vi "Poke-n-probe position.vi"(6 "Tries":i32=150, 7 "Goal":T1, 8 "error in":errorcluster, 9 "Speed":dbl=10.0, 10 "Zone":dbl=5.0 caption="mm", 11 "Location":string="Base") -> (0 "error out":errorcluster, 1 "Speed Out":dbl, 2 "Success":bool, 3 "Location Out":string="Base", 5 "Pose":T1)   [LabVIEW 2013]
uses:
  ROS/Code/Console/Servers/ServerSubs/(nist) Arm Globals.vi
panel:
  out "Array":dbl[][](array[numeric])
  out "Try":i32
  in  "stop":bool
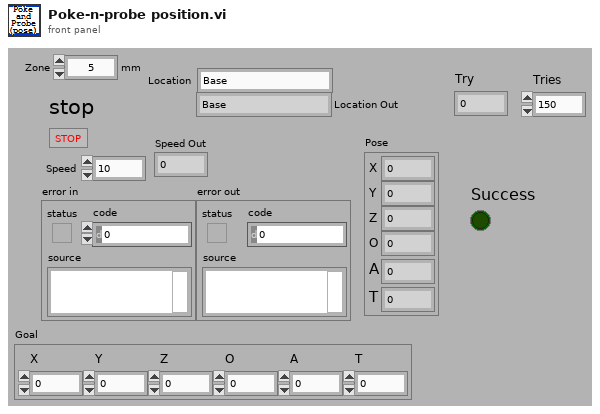
[diagram p1: front panel]
types:
  T1 = cluster{"X":dbl, "Y":dbl, "Z":dbl, "O":dbl, "A":dbl, "T":dbl}
  T2 = typedef "NI_Matrix.lvlib/RealMatrix.ctl" = dbl[][]
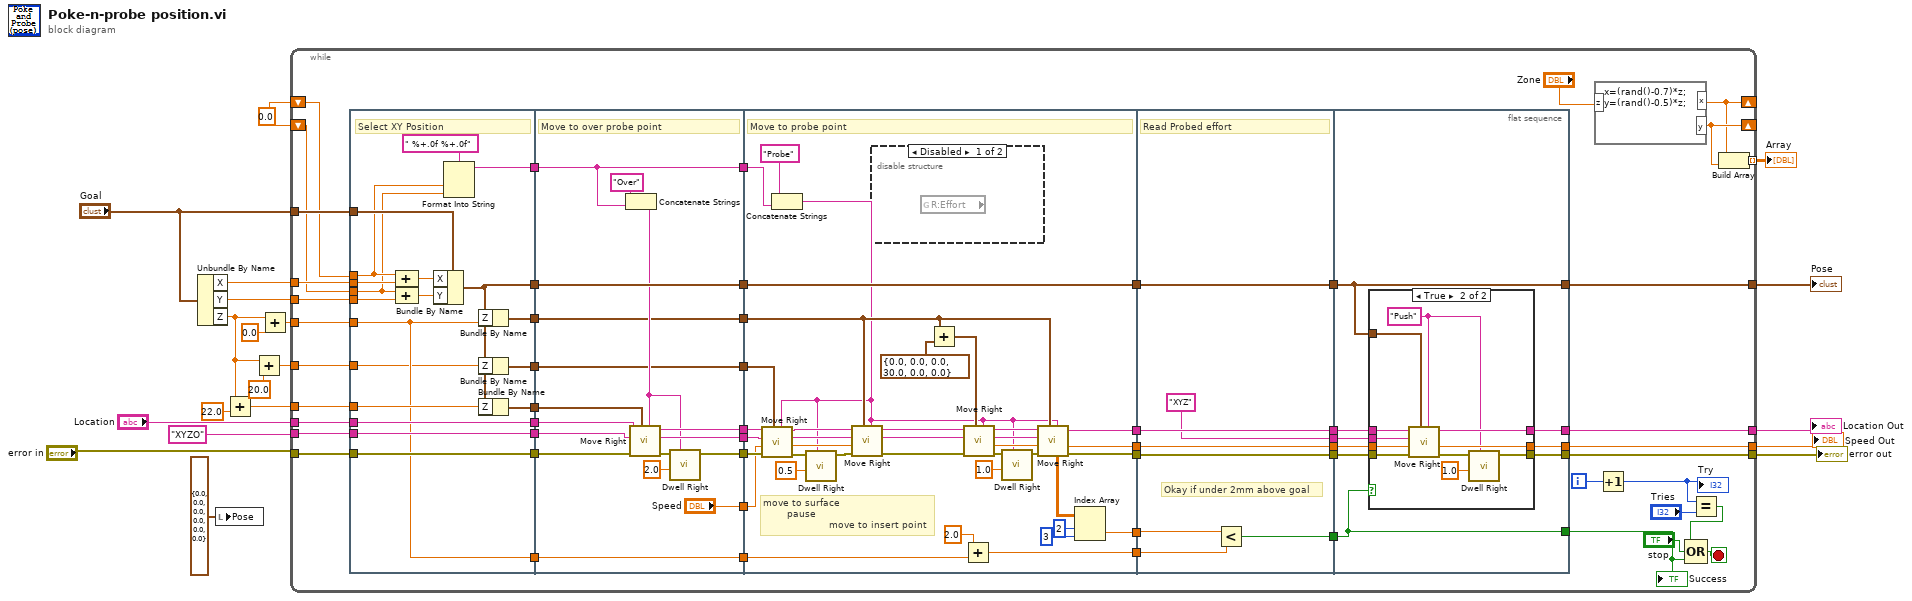
[diagram p0: block diagram]
diagram:
  w12 = 0.0
  n1 = Unbundle By Name("Goal") -> ("X"=w11:dbl, "Y"=w10:dbl, "Z"=w7:dbl)
  n2 = local write "Pose"(T1 {"X"=0.0, "Y"=0.0, "Z"=0.0, "O"=0.0, "A"=0.0, "T"=0.0} ("Pose")) -> ()
  n3 = Add(x=w7, y=22.0 ("x")) -> (x+y=w19:dbl)
  n4 = Add(x=w7, y=20.0) -> (x+y=w5:dbl)
  n5 = Add(x=w7, y=0.0) -> (x+y=w13:dbl)
  n6 = while {
    tunnel: "error in" -> [w71]
    tunnel: "Location" -> [w70]
    tunnel: "XYZO" ("Mask") -> [w69]
    tunnel: w19 -> [w68]
    tunnel: "Goal" -> [w67]
    tunnel: w10 -> [w66]
    tunnel: w11 -> [w65]
    tunnel: [w63] -> w18
    tunnel: [w62] -> w15
    tunnel: [w60] -> w17
    tunnel: [w59] -> w16
    tunnel: w13 -> [w46]
    shift-right: [w27] -> _
    shift-left: w12 -> [w42]
    shift-right: [w28] -> _
    shift-left: w12 -> [w41]
    tunnel: [w26] -> w9 mode=indexing
    tunnel: w5 -> [w25]
    i -> [w53]
    stop <- w57 stop-if-true
    n7 = flat-sequence {
      tunnel: w69 -> [w93]
      tunnel: w70 -> [w94]
      tunnel: w71 -> [w95]
      tunnel: [w95] -> w76
      tunnel: [w94] -> w75
      tunnel: [w93] -> w74
      tunnel: w68 -> [w92]
      tunnel: [w91] -> w73
      tunnel: [w79] -> w72
      tunnel: w67 -> [w90]
      tunnel: w66 -> [w81]
      tunnel: w65 -> [w89]
      tunnel: [w85] -> w55
      tunnel: w46 -> [w80]
      tunnel: [w84] -> w45
      tunnel: w42 -> [w83]
      tunnel: w41 -> [w82]
      tunnel: [w80] -> w32
      tunnel: w25 -> [w78]
      tunnel: [w77] -> w23
      tunnel: w76 -> [w112]
      tunnel: w75 -> [w111]
      tunnel: w74 -> [w109]
      tunnel: w73 -> [w110]
      tunnel: w72 -> [w107]
      tunnel: [w107] -> w40
      tunnel: [w106] -> w39
      tunnel: [w105] -> w38
      tunnel: [w104] -> w37
      tunnel: w55 -> [w101]
      tunnel: [w101] -> w36
      tunnel: [w99] -> w35
      tunnel: w45 -> [w99]
      tunnel: [w98] -> w33
      tunnel: w32 -> [w98]
      tunnel: [w97] -> w24
      tunnel: w23 -> [w97]
      tunnel: ["Speed"] -> w22
      tunnel: w40 -> [w141]
      tunnel: w39 -> [w131]
      tunnel: w38 -> [w130]
      tunnel: w37 -> [w129]
      tunnel: [w119] -> w64
      tunnel: [w141] -> w61
      tunnel: w36 -> [w148]
      tunnel: w35 -> [w136]
      tunnel: [w142] -> w44
      tunnel: [w139] -> w43
      tunnel: w33 -> [w117]
      tunnel: [w132] -> w31
      tunnel: w24 -> [w125]
      tunnel: w22 -> [w122]
      tunnel: [w115] -> w21
      tunnel: w64 -> [w155]
      tunnel: w61 -> [w154]
      tunnel: [w157] -> w51
      tunnel: [w156] -> w50
      tunnel: [w155] -> w49
      tunnel: [w154] -> w48
      tunnel: ["XYZ" ("Mask")] -> w47
      tunnel: w44 -> [w156]
      tunnel: w43 -> [w157]
      tunnel: w31 -> [w150]
      tunnel: [w152] -> w30
      tunnel: w21 -> [w151]
      tunnel: [w158] -> w62
      tunnel: [w162] -> w63
      tunnel: [w159] -> w58
      tunnel: [w160] -> w59
      tunnel: [w161] -> w60
      tunnel: w51 -> [w166]
      tunnel: w50 -> [w163]
      tunnel: w49 -> [w164]
      tunnel: w48 -> [w158]
      tunnel: w47 -> [w165]
      tunnel: w30 -> [w159]
      frame #0 {
        # "Select XY Position"
        n8 = Compound Arithmetic op=ADD(w83, w89) -> (w87:dbl)
        n9 = Compound Arithmetic op=ADD(w82, w81) -> (w86:dbl)
        n10 = Bundle By Name(cluster=w90, "X"=w87, "Y"=w86) -> (w79:T1)
        n11 = Format Into String(format string=" %+.0f %+.0f", w83, w82) -> (resulting string=w85:string)  [unwired: 2 in, 1 out]
        n12 = Bundle By Name(cluster=w79, "Z"=w80) -> (w84:T1)
        n13 = Bundle By Name(cluster=w79, "Z"=w78) -> (w77:T1)
        n14 = Bundle By Name(cluster=w79, "Z"=w92) -> (w91:T1)
      }
      frame #1 {
        # "Move to over probe point"
        n15 = Concatenate Strings("Over" ("string"), w101) -> (w100:string)
        n16 = call "Move Right.vi"("Label"=w100, "Goal"=w110, "error in"=w112, "Mask"=w109, "Location"=w111) -> ("error out"=w108:errorcluster, "Mask Out"=w105:string, "Location Out"=w106:string)  [unwired: 2 in, 2 out]
        n17 = call "Dwell Right.vi"("Label"=w100, "Wait Time"=2.0, "error in"=w108) -> ("error out"=w104:errorcluster)  [unwired: 8 in]
      }
      frame #2 {
        # "move to surface\n        pause\n                      move to insert point"
        # "Move to probe point"
        n18 = Concatenate Strings("Probe" ("Label"), w148) -> (w118:string)
        n19 = call "Move Right.vi"("Label"=w118, "Goal"=w125, "error in"=w129, "Speed"=w122, "Mask"=w130, "Location"=w131) -> ("error out"=w124:errorcluster, "Speed Out"=w126:dbl, "Mask Out"=w127:string, "Location Out"=w128:string)  [unwired: 1 in, 1 out]
        n20 = call "Dwell Right.vi"("Label"=w118, "Wait Time"=0.5, "error in"=w124) -> ("error out"=w123:errorcluster)  [unwired: 8 in]
        n21 = call "Move Right.vi"("Label"=w118, "Goal"=w136, "error in"=w123, "Speed"=w126, "Mask"=w127, "Location"=w128) -> ("error out"=w147:errorcluster, "Mask Out"=w144:string, "Location Out"=w146:string)  [unwired: 1 in, 2 out]
        n22 = disable-structure shown="Disabled" {
          frame Disabled {
            n23 = global read "(nist) Arm Globals.vi" "R:Effort"() -> ()  [unwired: 1 out]
          }
          frame Enabled {
          }
        }
        n24 = Add(x=w136, y=T1 {"X"=0.0, "Y"=0.0, "Z"=0.0, "O"=30.0, "A"=0.0, "T"=0.0}) -> (x+y=w145:T1)
        n25 = Add(x=2.0, y=w117) -> (x+y=w115:dbl)
        n26 = call "Move Right.vi"("Label"=w118, "Goal"=w145, "error in"=w147, "Mask"=w144, "Location"=w146) -> ("error out"=w121:errorcluster, "Speed Out"=w143:dbl, "Mask Out"=w138:string, "Location Out"=w140:string)  [unwired: 2 in, 1 out]
        n27 = call "Dwell Right.vi"("Label"=w118, "Wait Time"=1.0, "error in"=w121) -> ("error out"=w120:errorcluster)  [unwired: 8 in]
        n28 = call "Move Right.vi"("Label"=w118, "Goal"=w136, "error in"=w120, "Speed"=w143, "Mask"=w138, "Location"=w140) -> ("error out"=w119:errorcluster, "Speed Out"=w142:dbl, "Location Out"=w139:string, "Current"=w135:T2)  [unwired: 1 in, 1 out]
        n29 = Index Array(array=w135, index (row)=2, index (col)=3) -> (element=w132:dbl)
      }
      frame #3 {
        # "Okay if under 2mm above goal"
        # "Read Probed effort"
        n30 = Less?(x=w150, y=w151) -> (x < y?=w152:bool)
      }
      frame #4 {
        n31 = case shown="True" w159 {
          tunnel: w166 -> [w169 w178]
          tunnel: w165 -> [_ w177]
          tunnel: w164 -> [w167 w176]
          tunnel: w163 -> [w168 w175]
          tunnel: [w167 w174] -> w162
          tunnel: [w169 w173] -> w161
          tunnel: [w168 w172] -> w160
          tunnel: w158 -> [_ w170]
          frame False {
          }
          frame True {
            w171 = "Push" ("Label")
            n32 = call "Move Right.vi"("Label"=w171, "Goal"=w170, "error in"=w176, "Speed"=w175, "Mask"=w177, "Location"=w178) -> ("error out"=w179:errorcluster, "Speed Out"=w172:dbl, "Location Out"=w173:string)  [unwired: 1 in, 2 out]
            n33 = call "Dwell Right.vi"("Label"=w171, "Wait Time"=1.0, "error in"=w179) -> ("error out"=w174:errorcluster)  [unwired: 8 in]
          }
        }
      }
    }
    n34 = formula code="x=(rand()-0.7)*z;\ny=(rand()-0.5)*z;"("z"="Zone") -> ("x"=w27:dbl, "y"=w28:dbl)
    n35 = Increment(x=w53) -> (x+1=w29:i32)
    "Try" <- w29
    n36 = Equal?(x=w29, y="Tries") -> (x = y?=w52:bool)
    n37 = Compound Arithmetic op=OR(w52, "stop", w58) -> (w57:bool)
    n38 = Build Array(w27, w28) -> (w26:dbl[])
    "Success" <- w58
  }
  "error out" <- w18
  "Location Out" <- w17
  "Speed Out" <- w16
  "Pose" <- w15
  "Array" <- w9
